vi "Association Update Table for Spartan 5.0.vi"(8 "error in (no error)":errorcluster, 11 "Connection Refnum":T1) -> (0 "error out":errorcluster, 3 "Connection Refnum":T1)   [LabVIEW 2011]
uses:
  SI.LIB/ODBC/SQL Controls/Connection Refnum.ctl
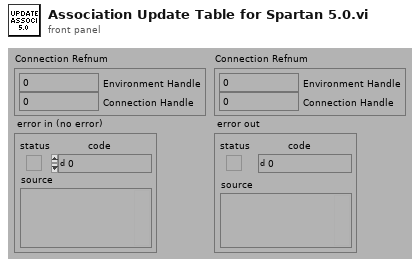
[diagram p1: front panel]
types:
  T1 = typedef "Connection Refnum.ctl" = cluster{"Environment Handle":i32, "Connection Handle":i32}
  T2 = typedef "Statement Refnum.ctl" = cluster{"Statement Handle":i32, "Parameter Number":u16}
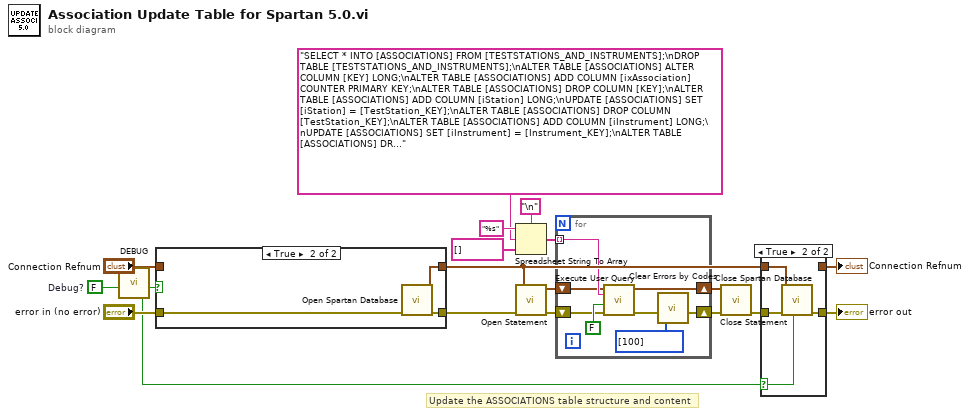
[diagram p0: block diagram]
diagram:
  w4 = FALSE  # Debug?
  # "Update the ASSOCIATIONS table structure and content"
  n1 = call "DEBUG.vi"("Dev DEBUG? (f)"=w4) -> ("DEBUG?"=w3:bool)  [unwired: 1 in, 5 out]
  n2 = case shown="True" w3 {
    tunnel: "Connection Refnum" -> [w20 _]
    tunnel: "error in (no error)" -> [w19 w23]
    tunnel: [w19 w22] -> w5
    tunnel: [w20 w21] -> w1
    frame False {
    }
    frame True {
      n3 = call "Open Spartan Database.vi"("error in (no error)"=w23) -> ("error out"=w22:errorcluster, "Connection Refnum"=w21:T1)  [unwired: 2 in, 7 out]
    }
  }
  n4 = Spreadsheet String To Array(delimiter (Tab)="\n", format string="%s", spreadsheet string="SELECT * INTO [ASSOCIATIONS] FROM [TESTSTATIONS_AND_INSTRUMENTS];\nDROP TABLE [TESTSTATIONS_AND_INSTRUMENTS];\nALTER TABLE [ASSOCIATIONS] ALTER COLUMN [KEY] LONG;\nALTER TABLE [ASSOCIATIONS] ADD COLUMN [ixAssociation] COUNTER PRIMARY KEY;\nALTER TABLE [ASSOCIATIONS] DROP COLUMN [KEY];\nALTER TABLE [ASSOCIATIONS] ADD COLUMN [iStation] LONG;\nUPDATE [ASSOCIATIONS] SET [iStation] = [TestStation_KEY];\nALTER TABLE [ASSOCIATIONS] DROP COLUMN [TestStation_KEY];\nALTER TABLE [ASSOCIATIONS] ADD COLUMN [iInstrument] LONG;\nUPDATE [ASSOCIATIONS] SET [iInstrument] = [Instrument_KEY];\nALTER TABLE [ASSOCIATIONS] DROP COLUMN [Instrument_KEY];" ("User Query"), array type (2D Dbl)=string[] []) -> (array=w17:string[])
  n5 = call "Open Statement.vi"("error in (no error)"=w5, "Connection Refnum"=w1) -> ("error out"=w13:errorcluster, "Statement Refnum"=w12:T2)  [unwired: 4 out]
  n6 = for {
    tunnel: w17 -> [w30] mode=indexing
    shift-right: [w27] -> w10
    shift-left: w12 -> [w29]
    shift-right: [w24] -> w11
    shift-left: w13 -> [w28]
    n7 = call "Execute User Query.vi"("error in (no error)"=w28, "Return Data? (f)"=FALSE, "User Query"=w30, "Statement Refnum"=w29) -> ("error out"=w25:errorcluster, "Statement Refnum"=w27:T2)  [unwired: 2 out]
    n8 = call "Clear Errors by Codes.vi"("Error Codes\nto Clear (Empty)"=i32[] [100] ("Error Codes\nto Clear (Empty)"), "error in (no error)"=w25) -> ("error out"=w24:errorcluster)  [unwired: 5 out]
  }
  n9 = call "Close Statement.vi"("error in (no error)"=w11, "Statement Refnum"=w10) -> ("error out"=w2:errorcluster)  [unwired: 5 out]
  n10 = case shown="True" w3 {
    selector: w3 -> [_ w34]
    tunnel: w2 -> [w33 w37]
    tunnel: w1 -> [w32 w36]
    tunnel: [w32 _] -> w9
    tunnel: [w33 w35] -> w8
    frame False {
    }
    frame True {
      n11 = call "Close Spartan Database.vi"("Force Close? (f)"=w34, "error in (no error)"=w37, "Connection Refnum"=w36) -> ("error out"=w35:errorcluster)  [unwired: 2 in, 6 out]
    }
  }
  "error out" <- w8
  "Connection Refnum" <- w9
